vi "Init_Test.vi"(8 "error in (no error)":errorcluster caption="entrée d'erreur (pas d'erreur)", 11 "Test (Default) en entrée":refnum<class "Sequencer_With_Firebase.lvclass">) -> (0 "error out":errorcluster caption="sortie d'erreur", 3 "Test (Default) en sortie":refnum<class "Sequencer_With_Firebase.lvclass">)   [LabVIEW 2020, in "Library Core.lvlib" / "Sequencer_With_Firebase.lvclass"]
uses:
  Sequencer_With_Firebase.lvclass
  C:/Users/ngarcin/OneDrive - Altyor/Standard TB/Class/Sequencer/Sequencer (Default)/Sequencer (Default).lvclass
  Commun VI/TypeDef/Actor Type.ctl
  Sequencer (Default)/Sequencer (Default).lvclass
  Sequencer_With_Firebase.lvclass/Sequencer_With_Firebase.ctl
  Commun VI/Library Commun.lvlib
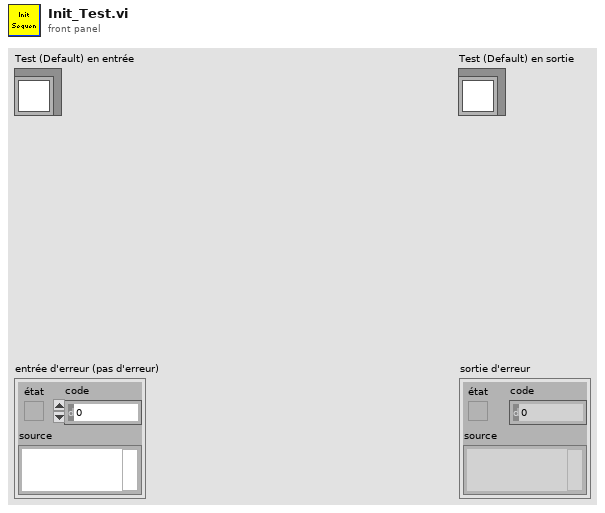
[diagram p1: front panel]
types:
  T1 = typedef "Library Commun.lvlib/Actor Type.ctl" = enum16{"Default", "Firebase", "Database"}
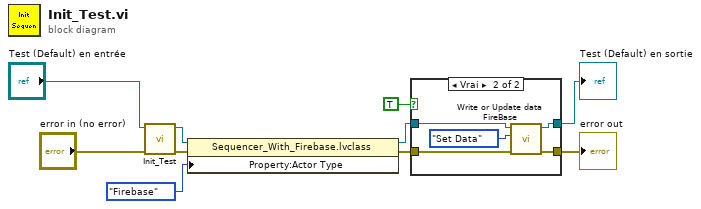
[diagram p0: block diagram]
diagram:
  n1 = call-parent "Init_Test.vi"("error in (no error)"="error in (no error)", "Test (Default) en entrée"="Test (Default) en entrée") -> ("error out"=w4:errorcluster, "Test (Default) en sortie"=w6:refnum<class "Sequencer_With_Firebase.lvclass">)  [unwired: 8 in]
  n2 = property class="Sequencer_With_Firebase.lvclass"(reference=w6, error in=w4, "Property:Actor Type"=Actor_Type."Firebase" ("Actor Type")) -> (reference out=w2:refnum<class "Sequencer_With_Firebase.lvclass">, error out=w3:errorcluster)
  n3 = case shown="Vrai" TRUE {
    tunnel: [w11 w16] -> w8
    tunnel: [w12 w15] -> w7
    tunnel: w3 -> [w12 w14]
    tunnel: w2 -> [w11 w13]
    frame False {
    }
    frame True {
      n4 = call-dynamic "Write or Update data FireBase.vi"("error in (no error)"=w14, "Function"=enum16{"Set Data", "Update Data"}."Set Data", "Sequencer IN"=w13) -> ("error out"=w15:errorcluster, "Sequencer Out"=w16:refnum<class "Sequencer_With_Firebase.lvclass">)  [unwired: 7 in]
    }
  }
  "error out" <- w7
  "Test (Default) en sortie" <- w8
